vi "VI Tree.vi"   [LabVIEW 2023, in "Error Manager.lvlib" / "NewErrorDialogueLoopQueue.lvlib"]
doc: "The library at a glance"
uses:
  NewErrorDialogueLoopQueue.lvlib
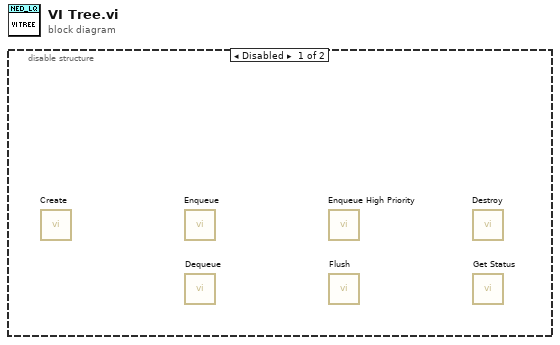
[diagram p0: block diagram]
diagram:
  n1 = disable-structure shown="Disabled" {
    frame Disabled {
      n2 = call "Create.vi"() -> ()  [unwired: 11 in, 1 out]
      n3 = call "Enqueue.vi"() -> ()  [unwired: 11 in, 1 out]
      n4 = call "Dequeue.vi"() -> ()  [unwired: 9 in, 3 out]
      n5 = call "Enqueue High Priority.vi"() -> ()  [unwired: 11 in, 1 out]
      n6 = call "Flush.vi"() -> ()  [unwired: 9 in, 3 out]
      n7 = call "Destroy.vi"() -> ()  [unwired: 9 in, 3 out]
      n8 = call "Get Status.vi"() -> ()  [unwired: 9 in, 3 out]
    }
    frame Enabled {
    }
  }
